vi "Create.vi"(8 "Error In":errorcluster, 11 "Session":refnum<class "Session.lvclass">) -> (0 "Error Out":errorcluster, 3 "Known Hosts":refnum<class "KnownHosts.lvclass">)   [LabVIEW 2017, in "LabSSH2.lvlib" / "KnownHosts.lvclass"]
uses:
  KnownHosts.lvclass
  Session/Session.lvclass
  KnownHosts.lvclass/KnownHosts.ctl
  <vilib>/Utility/error.llb/Error Cluster From Error Code.vi
  <vilib>/ErrorRing/Error Ring.xnode
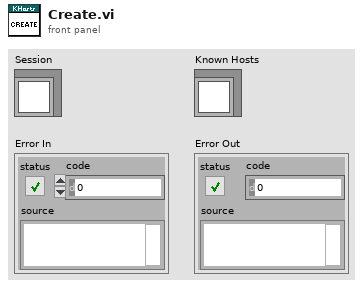
[diagram p1: front panel]
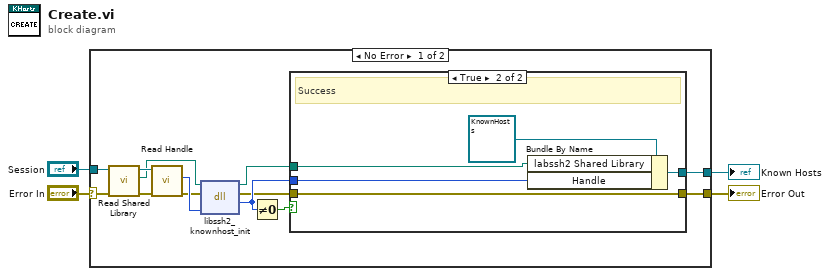
[diagram p0: block diagram]
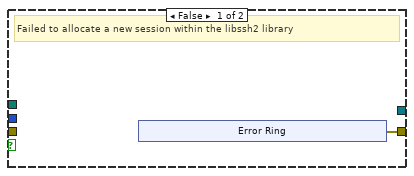
[diagram p2: hidden frame]
diagram:
  n1 = case shown="No Error" "Error In" {
    selector: "Error In" -> [w7 w28]
    tunnel: [w14 w28] -> w3
    tunnel: "Session" -> [w10 _]
    tunnel: [w12 _] -> w1
    frame No Error {
      n2 = call "Read Shared Library.vi"("Error In"=w7, "Session In"=w10) -> ("Erorr Out"=w8:errorcluster, "labssh2 Shared Library"=w5:path, "Session Out"=w9:refnum<class "Session.lvclass">)  [unwired: 7 in]
      n3 = call "Read Handle.vi"("Error In"=w8, "Session In"=w9) -> ("Erorr Out"=w6:errorcluster, "Handle"=w11:u64)  [unwired: 7 in, 1 out]
      n4 = dll-call lib="D:/Users/cfield/Code/Field R&D Services/SSH/LabSSH2/LabVIEW/trunk/src/LabSSH2/Private/labssh2.*" fn="libssh2_knownhost_init"(path in=w5, error in=w6, "session"=w11) -> (path out=w13:path, error out=w15:errorcluster, "KNOWNHOSTS"=w16:u64)  [unwired: 2 in]
      n5 = Not Equal To 0?(x=w16) -> (x != 0?=w17:bool)
      n6 = case shown="True" w17 {
        tunnel: w16 -> [_ w25]
        tunnel: w15 -> [_ w27]
        tunnel: [w18 w27] -> w14
        tunnel: w13 -> [_ w24]
        tunnel: [_ w23] -> w12
        frame False {
          # "Failed to allocate a new session within the libssh2 library"
          n7 = xnode "Error Ring"() -> ("error out"=w18:errorcluster)
        }
        frame True {
          # "Success"
          n8 = Bundle By Name(cluster=refnum<class "KnownHosts.lvclass"> refnum ("LabSSH2.lvlib:KnownHosts.lvclass"), "labssh2 Shared Library"=w24, "Handle"=w25) -> (w23:refnum<class "KnownHosts.lvclass">)
        }
      }
    }
    frame Error {
    }
  }
  "Error Out" <- w3
  "Known Hosts" <- w1
